vi "PlaceAckerman.vi"(9 "Poles":T2, 10 "B":T1, 11 "A":T1) -> (3 "K":T1)   [LabVIEW 2017]
uses:
  <vilib>/Analysis/Matrix/Datatypes/RealMatrix.ctl
  <vilib>/Analysis/Matrix/Datatypes/ComplexMatrix.ctl
  <vilib>/Analysis/7linalg.llb/Real Characteristic Polynomial.vi
  <vilib>/Analysis/7linalg.llb/Real Matrix Power.vi
  <vilib>/Analysis/baseanly.llb/Real A x B.vi
  <vilib>/Analysis/Matrix/Numeric/Conversions/Matrix To Array - CM.vi
  <vilib>/Analysis/baseanly.llb/Real Inverse Matrix.vi
  <vilib>/Analysis/Matrix/Numeric/Conversions/Array To Matrix - RA2.vi
  <vilib>/Analysis/Matrix/Numeric/Multiply/Multiply - RM,R.vi
  <vilib>/Analysis/Matrix/Numeric/Add/Add - RM,RM.vi
  <vilib>/Analysis/NI_AALPro.lvlib
  <vilib>/Analysis/Matrix/NI_Matrix.lvlib
  <vilib>/Analysis/NI_AALBase.lvlib
panel:
  out "Characteristic Polynomial":dbl[](array[numeric])
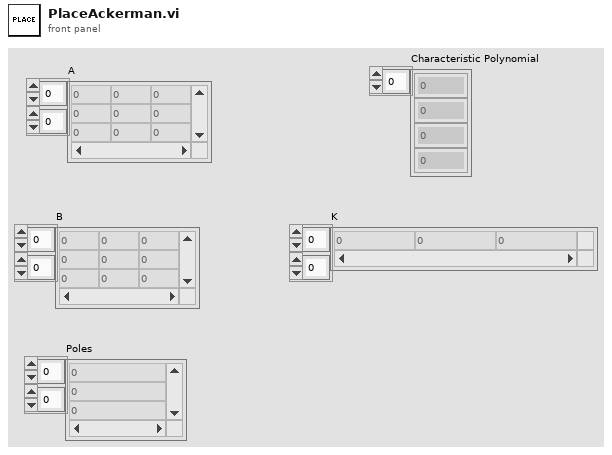
[diagram p1: front panel]
types:
  T1 = typedef "NI_Matrix.lvlib/RealMatrix.ctl" = dbl[][]
  T2 = typedef "NI_Matrix.lvlib/ComplexMatrix.ctl" = cdb[][]
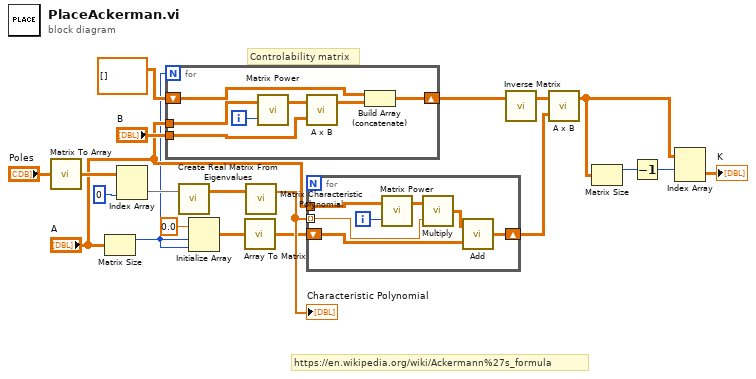
[diagram p0: block diagram]
diagram:
  # "Controlability matrix"
  # "https://en.wikipedia.org/wiki/Ackermann%27s_formula"
  n1 = call-poly <vilib>:"Matrix To Array.vi"("Complex Matrix"="Poles") -> ("Complex 2D Array"=w19:cdb[][])
  n2 = Matrix Size(0:"A") -> (1:w9:i32)  [unwired: 1 out]
  n3 = Index Array(array=w19, index (col)=0 ("disabled index (col)")) -> (element=w18:cdb[])  [unwired: 1 in]
  n4 = for {
    N: w9 -> [_]
    tunnel: "A" -> [w26]
    tunnel: "B" -> [w24]
    shift-right: [w23] -> w12
    shift-left: T1 [] ("A x B") -> [w22]
    i -> [w27]
    n5 = call-poly <vilib>:"Matrix Power.vi"("n"=w27, "Input Matrix"=w26) -> ("Matrix Power"=w25:T1)  [unwired: 1 out]
    n6 = call-poly <vilib>:"A x B.vi"("B"=w24, "A"=w25) -> ("A x B"=w21:T1)  [unwired: 1 out]
    n7 = Build Array (concatenate)(w22, w21) -> (w23:T1)
  }
  n8 = call <vilib>:"Create Real Matrix From Eigenvalues.vi"("Eigenvalues"=w18) -> ("Matrix"=w16:T1)  [unwired: 1 in, 1 out]
  n9 = Initialize Array(0.0 ("element"), w9, w9) -> (w8:dbl[][])
  n10 = call-poly <vilib>:"Array To Matrix.vi"("Real 2D Array"=w8) -> ("Real Matrix"=w7:T1)
  n11 = call-poly <vilib>:"Matrix Characteristic Polynomial.vi"("Input Matrix"=w16) -> ("Characteristic Polynomial"=w15:dbl[])  [unwired: 1 in, 1 out]
  "Characteristic Polynomial" <- w15
  n12 = for {
    tunnel: w15 -> [w29] mode=indexing
    tunnel: "A" -> [w33]
    shift-right: [w32] -> w6
    shift-left: w7 -> [w31]
    i -> [w34]
    n13 = call-poly <vilib>:"Matrix Power.vi"("n"=w34, "Input Matrix"=w33) -> ("Matrix Power"=w30:T1)  [unwired: 1 out]
    n14 = call-poly <vilib>:"Multiply.vi"("Real Scalar c"=w29, "Real Matrix A"=w30) -> ("A * c"=w28:T1)
    n15 = call-poly <vilib>:"Add.vi"("Real Matrix B"=w31, "Real Matrix A"=w28) -> ("A + B"=w32:T1)
  }
  n16 = call-poly <vilib>:"Inverse Matrix.vi"("Input Matrix"=w12) -> ("Inverse Matrix"=w5:T1)  [unwired: 1 in, 1 out]
  n17 = call-poly <vilib>:"A x B.vi"("B"=w6, "A"=w5) -> ("A x B"=w4:T1)  [unwired: 1 out]
  n18 = Matrix Size(0:w4) -> (1:w2:i32)  [unwired: 1 out]
  n19 = Decrement(x=w2) -> (x-1=w1:i32)
  n20 = Index Array(array=w4, index (row)=w1) -> (element=→"K":T1)  [unwired: 1 in]
